vi "configuration UI.vi"() -> ()   [LabVIEW 2013, in "UI Reference editor node.lvclass"]
uses:
  UI Reference editor node.lvclass
  <vilib>/CEF_TreeControl/Node/NodeRef.ctl
  <vilib>/CEF_TreeControl/Node/NISE_CEF_Node.lvclass
  <vilib>/NI/AMC/Message Queue.ctl
  <vilib>/NI/AMC/Message.ctl
  <vilib>/NI/Tools/Keyed Array/KeyedArray.ctl
  <vilib>/CEF_TreeControl/Node/UserEventRef.ctl
  <vilib>/CEF_TreeControl/Controls/EventCluster.ctl
  module/configuration/UI Reference configuration.lvclass
  <vilib>/NI/Module Execution Interface/Engine Configuration/engine configuration.lvclass
  <vilib>/NI/Tag Bus Data Framework/Configuration Editor/Classes/Engine Parent/Engine Parent Editor Node.lvclass
  <vilib>/NI/Tag Bus/tag/tag descriptor.lvclass
  <vilib>/NI/Tag Bus/tag/Data Type.ctl
  <vilib>/NI/Tag Bus/tag/tag descriptor.lvclass/tag descriptor.ctl
  <vilib>/NI/Tag Bus Module Framework/root configuration/TBM configuration.lvclass/TBM configuration.ctl
  module/configuration/UI Reference configuration.lvclass/UI Reference configuration.ctl
  <vilib>/NI/Tag Bus/tag/write tag name.vi
  <vilib>/NI/Tag Bus/tag/write data type.vi
  <vilib>/NI/Tag Bus Module Framework/root configuration/Read instance name.vi
  module/configuration/Read VI name.vi
  <vilib>/NI/Tag Bus Data Framework/Configuration Editor/Classes/Module editor node/Read Module Configuration.vi
  <vilib>/NI/Tag Bus Module Framework/root configuration/create GUID.vi
  <vilib>/NI/Tag Bus Module Framework/root configuration/TBM configuration.lvclass
  <vilib>/NI/Tag Bus Module Framework/module configuration/TBM module configuration.lvclass
  <vilib>/NI/Tag Bus Module Framework/channel/TBM channel.lvclass
  <vilib>/CEF_TreeControl/NISE_CEF_TreeControl.lvlib
  <vilib>/NI/Tag Bus Data Framework/Configuration Editor/Classes/Module editor node/module editor node.lvclass
  <vilib>/NI/Tools/Keyed Array/Tools_KeyedArray.lvlib
  <vilib>/NI/AMC/AMC.lvlib
panel:
  in  "Tab Control":enum32{"Static Configuration"}(tab)
  in  "autogen":bool
  in  "browse":bool
  out "UI to Load":string
  in  "hidden_remove":bool
  in  "hidden_settings":bool
  in  "hidden_Add":bool
  in  "Remove Button":bool
  in  "Add Button":bool
  in  "channel":i32(listbox)
  in  "settings":bool
  in  "user event":T1
  in  "main queue":T2
  in  "node ref":T3
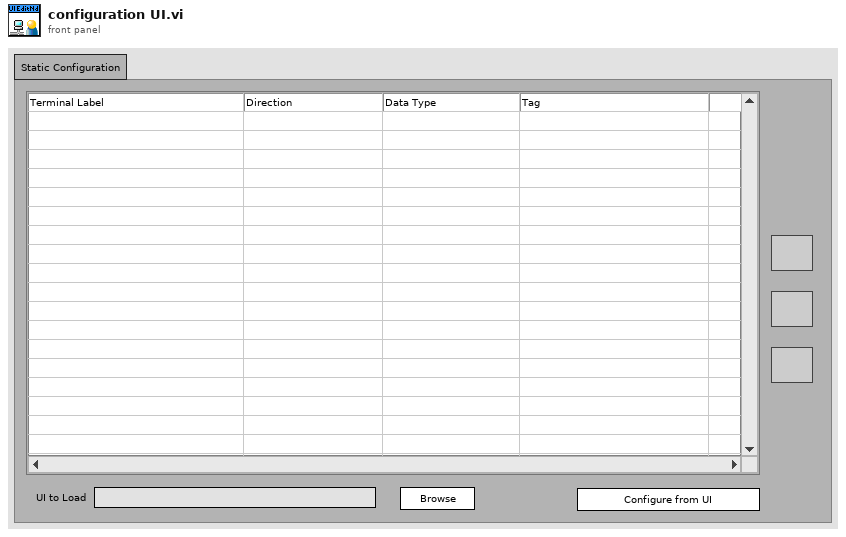
[diagram p1: front panel]
types:
  T1 = typedef "NISE_CEF_Node.lvclass/UserEventRef.ctl" = refnum<user-event>
  T2 = typedef "AMC.lvlib/Message Queue.ctl" = refnum<queue>
  T3 = typedef "NISE_CEF_Node.lvclass/NodeRef.ctl" = refnum<data-value>
  T4 = typedef "tag bus.lvlib/tag descriptor.lvclass/Data Type.ctl" = enum16{"Double", "Single", "I64", "I32", "I16", "I8", "U64", "U32", "U16", "U8", "Boolean", "String", "Array of Double", "Array of Single", "Array of I64", "Array of I32", "Array of I16", "Array of I8", "Array of U64", "Array of U32", "Array of U16", "Array of U8", "Array of Boolean", "Array of String"}
  T5 = typedef "NISE_CEF_TreeControl.lvlib/EventCluster.ctl" = cluster{"command":string, "data":string}
  T6 = typedef "UI Reference editor node.lvclass/table line.ctl" = cluster{"channel":refnum<class "TBM channel.lvclass">, "tag name":string}
  T7 = typedef "LVPoint32TypeDef.ctl" = cluster{"Horizontal":i32, "Vertical":i32}
  T8 = typedef "LVRowAndColumnTypeDef.ctl" = cluster{"Row":i32, "Column":i32}
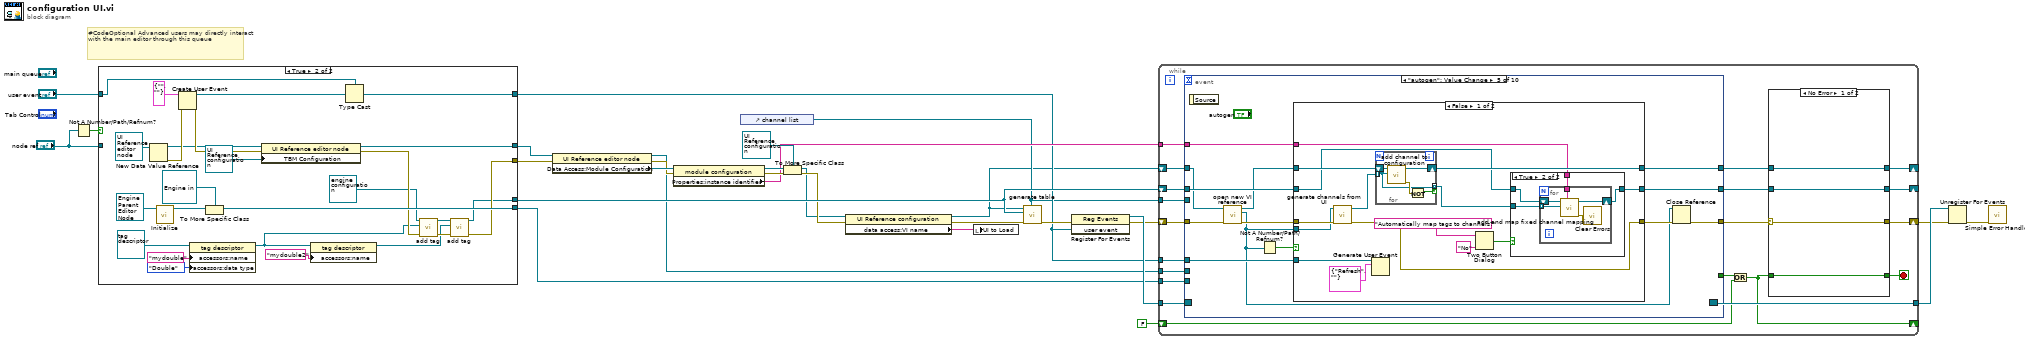
[diagram p0: block diagram]
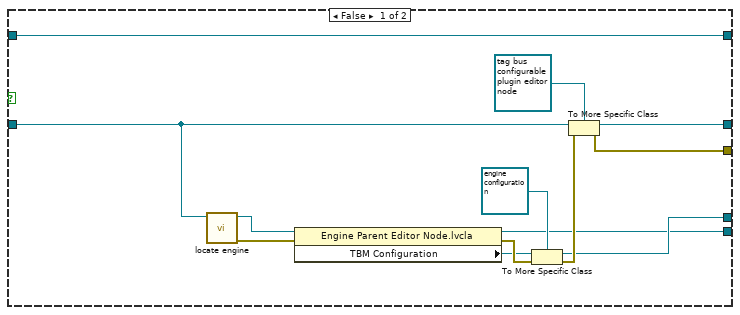
[diagram p2: hidden frame]
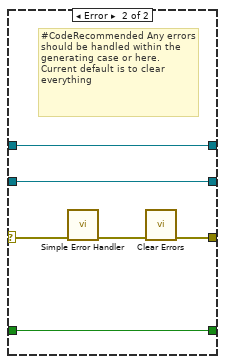
[diagram p3: hidden frame]
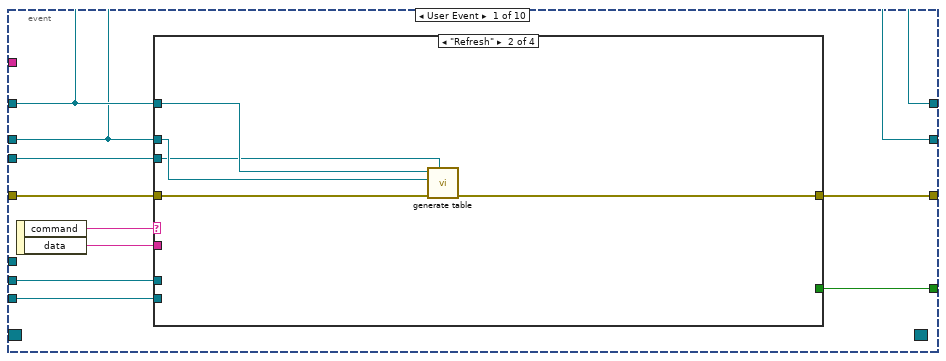
[diagram p4: hidden frame]
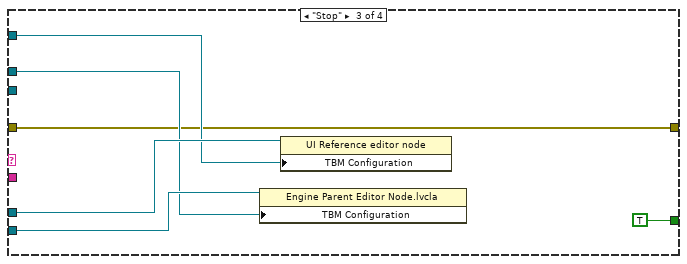
[diagram p6: hidden frame]
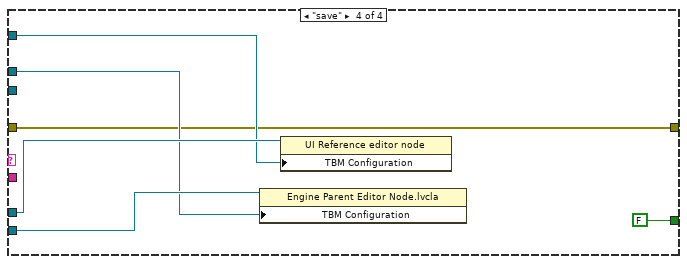
[diagram p7: hidden frame]
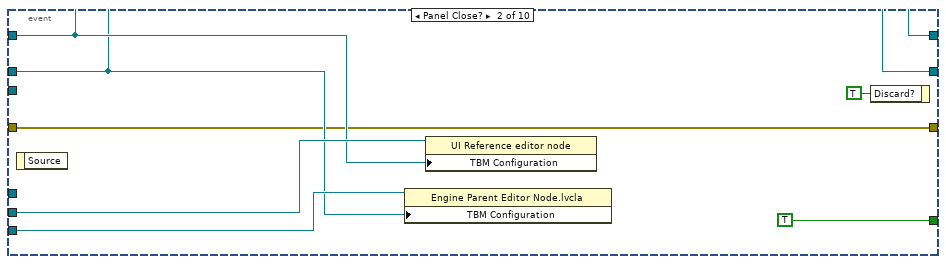
[diagram p8: hidden frame]
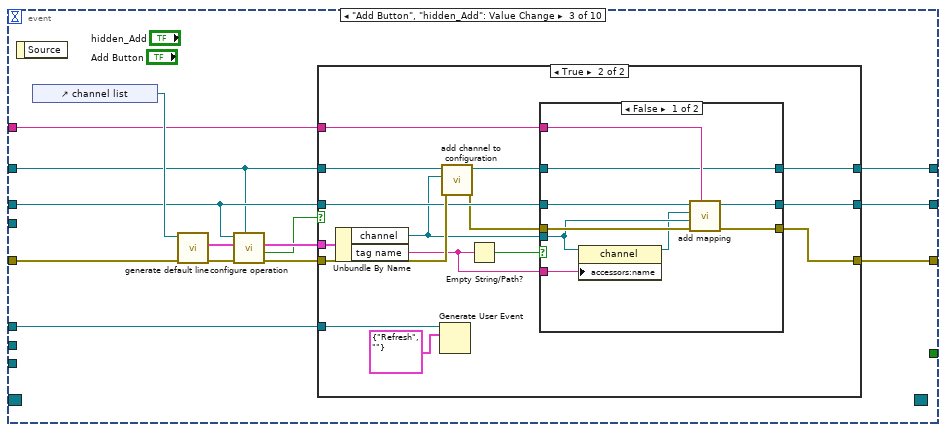
[diagram p9: hidden frame]
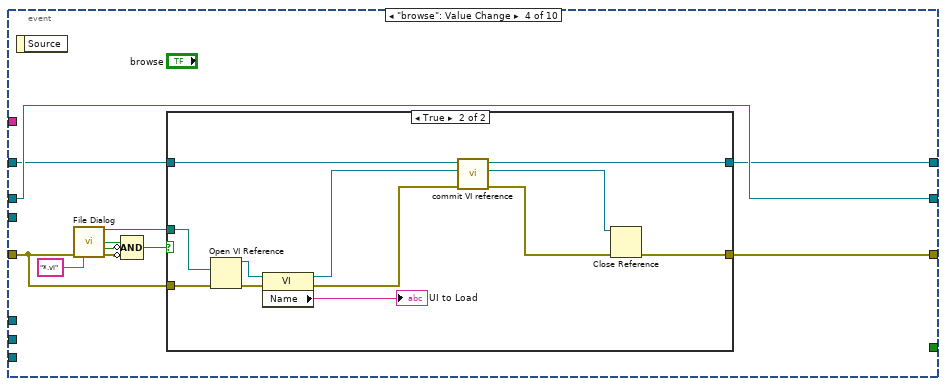
[diagram p12: hidden frame]
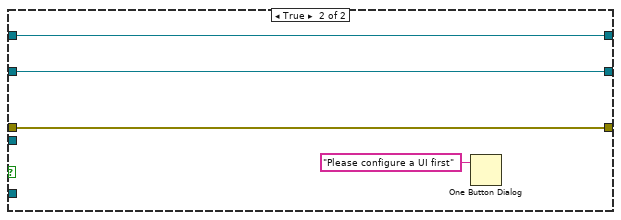
[diagram p15: hidden frame]
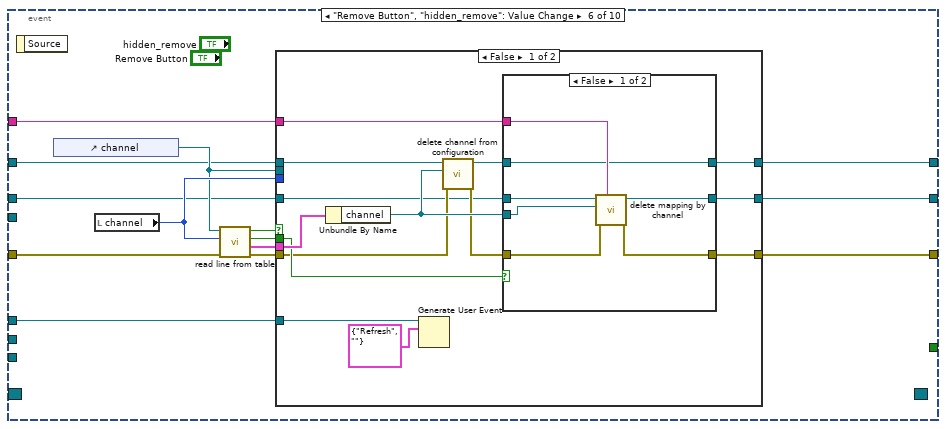
[diagram p16: hidden frame]
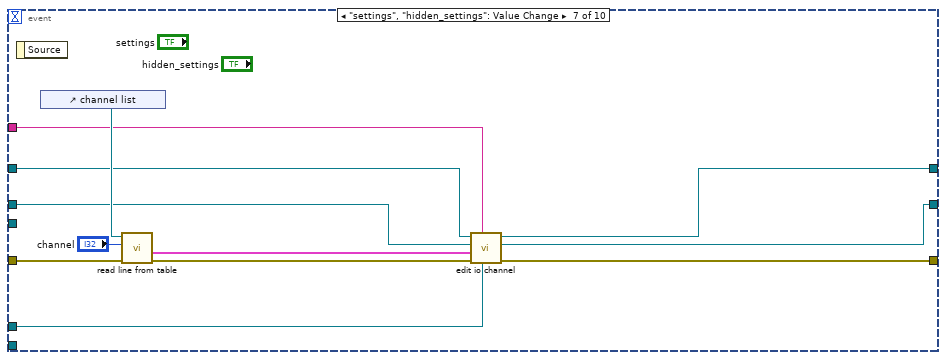
[diagram p19: hidden frame]
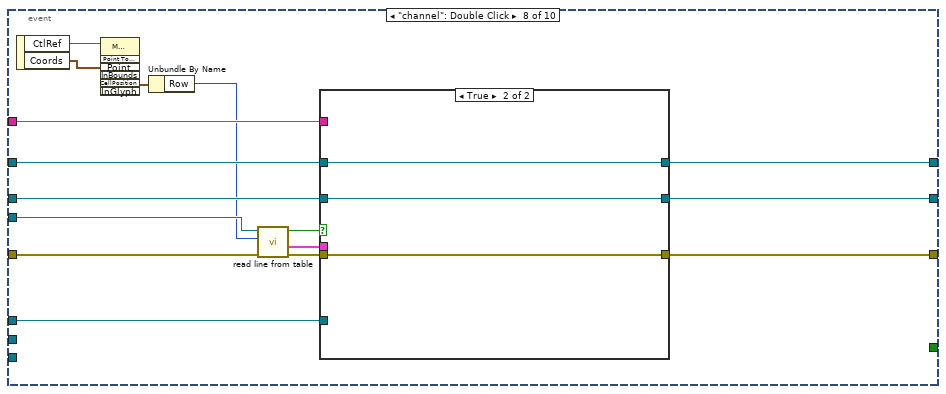
[diagram p20: hidden frame]
diagram:
  # "#CodeOptional Advanced users may directly interact with the main editor through this queue"
  n1 = Not A Number/Path/Refnum?(number/path/refnum="node ref") -> (NaN/Path/Refnum?=w19:bool)
  n2 = case shown="True" w19 {
    tunnel: "user event" -> [w41 w43]
    tunnel: [w41 w44] -> w6
    tunnel: "node ref" -> [w39 _]
    tunnel: [w38 w61] -> w12
    tunnel: [w37 w48] -> w17
    tunnel: [w30 w47] -> w14
    tunnel: [w29 w58] -> w8
    frame False {
      n3 = call <vilib>:"locate engine.vi"("component"=w39) -> ("error out"=w34:errorcluster, "engine"=w36:refnum<data-value>)  [unwired: 9 in]
      n4 = property class="Engine Parent Editor Node.lvcla"(reference=w36, error in=w34) -> (reference out=w29:refnum<data-value>, error out=w33:errorcluster, "TBM Configuration"=w32:refnum<class "TBM configuration.lvclass">)
      n5 = To More Specific Class(target class=refnum<class "engine configuration.lvclass"> refnum ("engine configuration.lvclass"), reference=w32, error in=w33) -> (specific class reference=w30:refnum<class "engine configuration.lvclass">, error out=w31:errorcluster)
      n6 = To More Specific Class(target class=refnum<data-value> refnum ("data value reference"), reference=w39, error in=w31) -> (specific class reference=w38:refnum<data-value>, error out=w37:errorcluster)
    }
    frame True {
      n7 = New Data Value Reference(data value=refnum<class "UI Reference editor node.lvclass"> refnum ("tag bus configurable plugin editor node")) -> (data value reference=w60:refnum<data-value>, error out=w63:errorcluster)  [unwired: 1 in]
      n8 = call-dynamic "Initialize.vi"("Engine in"=refnum<class "Engine Parent Editor Node.lvclass"> refnum) -> ("data value reference"=w59:T3)  [unwired: 8 in, 2 out]
      n9 = Create User Event(user event datatype=T5 {"command"="", "data"=""} ("event data"), error in=w63) -> (user event=w66:refnum<user-event>, error out=w62:errorcluster)
      n10 = property class="tag descriptor"(reference=refnum<class "tag descriptor.lvclass"> refnum ("tag descriptor"), "accessors:name"="mydouble" ("name"), "accessors:data type"=Data_Type."Double" ("data type")) -> (reference out=w45:refnum<class "tag descriptor.lvclass">)  [unwired: 1 in, 1 out]
      n11 = To More Specific Class(target class=refnum<data-value> refnum ("data value reference"), reference=w59) -> (specific class reference=w58:refnum<data-value>)  [unwired: 1 in, 1 out]
      n12 = property class="UI Reference editor node"(reference=w60, error in=w62, "TBM Configuration"=refnum<class "UI Reference configuration.lvclass"> refnum ("tag bus configurable plugin module configuration")) -> (reference out=w61:refnum<data-value>, error out=w52:errorcluster)
      n13 = property class="tag descriptor"(reference=w45, "accessors:name"="mydouble2" ("name")) -> (reference out=w46:refnum<class "tag descriptor.lvclass">)  [unwired: 1 in, 1 out]
      n14 = Type Cast(type=w43, x=w66) -> (*(type *) &x=w44:T1)
      n15 = call <vilib>:"add tag.vi"("error in"=w52, "tag descriptor"=w45, "engine configuration in"=refnum<class "engine configuration.lvclass"> refnum ("Engine Configuration")) -> ("error out"=w50:errorcluster, "engine configuration out"=w49:refnum<class "engine configuration.lvclass">)  [unwired: 7 in]
      n16 = call <vilib>:"add tag.vi"("error in"=w50, "tag descriptor"=w46, "engine configuration in"=w49) -> ("error out"=w48:errorcluster, "engine configuration out"=w47:refnum<class "engine configuration.lvclass">)  [unwired: 7 in]
    }
  }
  n17 = property class="UI Reference editor node"(reference=w12, error in=w17) -> (reference out=w9:refnum<data-value>, error out=w22:errorcluster, "Data Access:Module Configuration"=w23:refnum<class "TBM module configuration.lvclass">)
  n18 = property class="module configuration"(reference=w23, error in=w22) -> (reference out=w20:refnum<class "TBM module configuration.lvclass">, error out=w21:errorcluster, "Properties:instance identifier"=w16:string)
  n19 = control-ref of="channel list"() -> (w5:refnum<vi>)
  n20 = To More Specific Class(target class=refnum<class "UI Reference configuration.lvclass"> refnum ("tag bus configurable plugin module configuration"), reference=w20, error in=w21) -> (specific class reference=w3:refnum<class "UI Reference configuration.lvclass">, error out=w13:errorcluster)
  n21 = property class="UI Reference configuration"(reference=w3, error in=w13) -> (reference out=w2:refnum<class "UI Reference configuration.lvclass">, error out=w4:errorcluster, "data access:VI name"=w1:string)
  n22 = local write "UI to Load"(w1) -> ()
  n23 = call "generate table.vi"("table"=w5, "error in"=w4, "engine configuration"=w14, "tag bus configurable plugin module configuration"=w2) -> ("error out"=w11:errorcluster)  [unwired: 7 in]
  n24 = register-events(error in=w11, w6) -> (reference out=w28:refnum<event-registration>, error out=w10:errorcluster)  [unwired: 1 in]
  n25 = while {
    tunnel: w28 -> [w87]
    tunnel: [w86] -> w27
    shift-right: [w80] -> w26
    shift-left: w10 -> [w85]
    shift-right: [w82] -> _
    shift-left: FALSE -> [w81]
    shift-right: [w76] -> _
    shift-left: w2 -> [w79]
    shift-right: [w77] -> _
    shift-left: w14 -> [w78]
    tunnel: w16 -> [w75]
    tunnel: w9 -> [w72]
    tunnel: w8 -> [w71]
    tunnel: w6 -> [w70]
    tunnel: w5 -> [w68]
    stop <- w84 stop-if-true
    n26 = event shown="[4] \"autogen\": Value Change" {
      selector: w87 -> [_ _ _ _ _ _ _ _ _ _]
      dyn-events: [_ _ _ _ _ _ _ _ _ _] -> w86
      timeout: _ -> [_ _ _ _ _ _ _ _ _ _]
      tunnel: [w107 TRUE _ _ _ _ _ _ _ _] -> w83
      tunnel: [w99 w127 w146 w179 w203 w262 w300 w316 w330 w365] -> w69
      tunnel: w85 -> [w100 w127 w145 w181 w207 w261 w301 w317 w348 w364]
      tunnel: w79 -> [w103 w129 w133 w178 w206 w257 w294 w312 w337 w369]
      tunnel: w78 -> [w102 w128 w134 w187 w212 w256 w295 w313 w333 w368]
      tunnel: [w102 w128 w139 w187 w213 w251 w292 w310 w334 w366] -> w74
      tunnel: [w103 w129 w138 w177 w211 w250 w293 w311 w335 w367] -> w73
      tunnel: w75 -> [_ _ w137 _ w209 w252 w291 w309 _ _]
      tunnel: w72 -> [w105 w131 _ _ _ _ _ _ _ _]
      tunnel: w71 -> [w104 w130 _ _ _ _ _ _ _ _]
      tunnel: w70 -> [_ _ w135 _ w208 w249 w290 w308 _ _]
      tunnel: w68 -> [w98 _ _ _ _ _ _ w307 _ _]
      event User Event {
        n27 = event-data() -> ("command"=w106:string, "data"=w101:string)  [unwired: 1 in]
        n28 = case shown="\"Refresh\"" w106 {
          tunnel: [_ _ TRUE FALSE] -> w107
          tunnel: w105 -> [_ _ w118 w124]
          tunnel: w104 -> [_ _ w117 w123]
          tunnel: w103 -> [_ w113 w116 w122]
          tunnel: w102 -> [_ w112 w115 w121]
          tunnel: w101 -> [_ _ _ _]
          tunnel: w100 -> [w108 w111 w114 w120]
          tunnel: [w108 w110 w114 w120] -> w99
          tunnel: w98 -> [_ w109 _ _]
          frame Default {
          }
          frame "Refresh" {
            n29 = call "generate table.vi"("table"=w109, "error in"=w111, "engine configuration"=w112, "tag bus configurable plugin module configuration"=w113) -> ("error out"=w110:errorcluster)  [unwired: 7 in]
          }
          frame "Stop" {
            n30 = property class="Engine Parent Editor Node.lvcla"(reference=w117, "TBM Configuration"=w115) -> ()  [unwired: 1 in, 2 out]
            n31 = property class="UI Reference editor node"(reference=w118, "TBM Configuration"=w116) -> ()  [unwired: 1 in, 2 out]
          }
          frame "save" {
            n32 = property class="Engine Parent Editor Node.lvcla"(reference=w123, "TBM Configuration"=w121) -> ()  [unwired: 1 in, 2 out]
            n33 = property class="UI Reference editor node"(reference=w124, "TBM Configuration"=w122) -> ()  [unwired: 1 in, 2 out]
          }
        }
      }
      event Panel Close? {
        n34 = event-data() -> ()  [unwired: 1 in, 1 out]
        n35 = property class="Engine Parent Editor Node.lvcla"(reference=w130, "TBM Configuration"=w128) -> ()  [unwired: 1 in, 2 out]
        n36 = property class="UI Reference editor node"(reference=w131, "TBM Configuration"=w129) -> ()  [unwired: 1 in, 2 out]
        n37 = event-data("Discard?"=TRUE) -> ()  [unwired: 1 in, 1 out]
      }
      event "Add Button", "hidden_Add": Value Change {
        n38 = event-data() -> ()  [unwired: 1 in, 1 out]
        n39 = control-ref of="channel list"() -> (w144:refnum<vi>)
        n40 = call "generate default line.vi"("error in"=w145, "operations table"=w144) -> ("error out"=w142:errorcluster, "line"=w143:T6)  [unwired: 8 in]
        n41 = call "configure operation.vi"("tag bus configurable plugin module configuration"=w133, "error in"=w142, "line item in"=w143, "engine configuration"=w134) -> ("error out"=w140:errorcluster, "success"=w136:bool, "line item out"=w141:T6)  [unwired: 4 in, 1 out]
        n42 = case shown="True" w136 {
          tunnel: [w149 w152] -> w146
          tunnel: w140 -> [w149 w162]
          tunnel: w134 -> [w148 w160]
          tunnel: w141 -> [_ w163]
          tunnel: w133 -> [w147 w164]
          tunnel: [w148 w159] -> w139
          tunnel: [w147 w153] -> w138
          tunnel: w137 -> [_ w156]
          tunnel: w135 -> [_ w151]
          frame False {
          }
          frame True {
            n43 = Unbundle By Name(w163) -> ("channel"=w157:refnum<class "TBM channel.lvclass">, "tag name"=w155:string)
            n44 = Generate User Event(user event=w151, event data cluster=T5 {"command"="Refresh", "data"=""} ("event data")) -> ()  [unwired: 2 in, 2 out]
            n45 = call "add channel to configuration.vi"("error in"=w162, "channel"=w157, "UI Reference configuration in"=w164) -> ("error out"=w158:errorcluster, "UI Reference configuration out"=w154:refnum<class "UI Reference configuration.lvclass">)  [unwired: 7 in]
            n46 = Empty String/Path?(string/path=w155) -> (empty?=w161:bool)
            n47 = case shown="False" w161 {
              tunnel: w160 -> [w173 w176]
              tunnel: [w172 w176] -> w159
              tunnel: w158 -> [w171 w175]
              tunnel: w157 -> [w169 _]
              tunnel: w156 -> [w170 _]
              tunnel: w155 -> [w168 _]
              tunnel: [w166 w175] -> w152
              tunnel: w154 -> [w165 w174]
              tunnel: [w165 w174] -> w153
              frame False {
                n48 = property class="channel"(reference=w169, "accessors:name"=w168) -> (reference out=w167:refnum<class "TBM channel.lvclass">)  [unwired: 1 in, 1 out]
                n49 = call <vilib>:"add mapping.vi"("owner ID"=w170, "error in"=w171, "channel"=w169, "tag descriptor"=w167, "engine configuration"=w173) -> ("error out"=w166:errorcluster, "engine configuration out"=w172:refnum<class "engine configuration.lvclass">)  [unwired: 5 in]
              }
              frame True {
              }
            }
          }
        }
      }
      event "browse": Value Change {
        n50 = event-data() -> ()  [unwired: 1 in, 1 out]
        n51 = call "File Dialog"("error in"=w181, "pattern (all files)"="*.vi") -> ("selected path"=w180:path, "exists"=w185:bool, "cancelled"=w184:bool, "error out"=w183:errorcluster)  [unwired: 10 in]
        n52 = Compound Arithmetic op=AND(w185, invert w184, invert w183) -> (w182:bool)
        n53 = case shown="True" w182 {
          tunnel: w181 -> [w189 w201]
          tunnel: w180 -> [_ w200]
          tunnel: [w189 w193] -> w179
          tunnel: w178 -> [w188 w196]
          tunnel: [w188 w195] -> w177
          frame False {
          }
          frame True {
            n54 = Open VI Reference(vi path=w200, error in (no error)=w201) -> (vi reference=w198:refnum<vi>, error out=w199:errorcluster)  [unwired: 4 in]
            n55 = property class="VI"(reference=w198, error in=w199) -> (reference out=w190:refnum<vi>, error out=w191:errorcluster, "Name"=→"UI to Load":string)
            n56 = call "commit VI reference.vi"("error in"=w191, "VI Refnum in"=w190, "UI Reference configuration in"=w196) -> ("error out"=w194:errorcluster, "VI Refnum out"=w192:refnum<vi>, "UI Reference configuration out"=w195:refnum<class "UI Reference configuration.lvclass">)  [unwired: 6 in]
            n57 = Close Reference(reference=w192, error in (no error)=w194) -> (error out=w193:errorcluster)
          }
        }
      }
      event "autogen": Value Change {
        n58 = event-data() -> ()  [unwired: 1 in, 1 out]
        n59 = call "open new VI reference.vi"("error in"=w207, "UI Reference configuration in"=w206) -> ("error out"=w204:errorcluster, "VI Refnum"=w202:refnum<vi>, "UI Reference configuration out"=w205:refnum<class "UI Reference configuration.lvclass">)  [unwired: 7 in]
        n60 = Not A Number/Path/Refnum?(number/path/refnum=w202) -> (NaN/Path/Refnum?=w214:bool)
        n61 = case shown="False" w214 {
          tunnel: w204 -> [w229 w246]
          tunnel: w205 -> [w227 w247]
          tunnel: [w220 w248] -> w213
          tunnel: w212 -> [w221 w248]
          tunnel: [w222 w247] -> w211
          tunnel: [w218 w246] -> w210
          tunnel: w202 -> [w228 _]
          tunnel: w209 -> [w217 _]
          tunnel: w208 -> [w215 _]
          frame False {
            n62 = call "generate channels from UI.vi"("error in"=w229, "VI Refnum"=w228) -> ("error out"=w218:errorcluster, "channels"=w226:refnum<class "TBM channel.lvclass">[])  [unwired: 8 in]
            n63 = Generate User Event(user event=w215, event data cluster=T5 {"command"="Refresh", "data"=""} ("event data")) -> ()  [unwired: 2 in, 2 out]
            n64 = for {
              tunnel: w226 -> [w241] mode=indexing
              shift-right: [w243] -> w222
              shift-left: w227 -> [w244]
              tunnel: [w241] -> w219 mode=indexing if=w240
              n65 = call "add channel to configuration.vi"("channel"=w241, "UI Reference configuration in"=w244) -> ("error out"=w242:errorcluster, "UI Reference configuration out"=w243:refnum<class "UI Reference configuration.lvclass">)  [unwired: 8 in]
              n66 = Not(x=w242) -> (.not. x?=w240:bool)
            }
            n67 = Two Button Dialog(message="Automatically map tags to channels?", 1:"No" ("F button name (\"Cancel\")")) -> (T button?=w223:bool)  [unwired: 1 in]
            n68 = case shown="True" w223 {
              tunnel: w221 -> [w230 w234]
              tunnel: [w230 w233] -> w220
              tunnel: w219 -> [_ w232]
              tunnel: w217 -> [_ w231]
              frame False {
              }
              frame True {
                n69 = for {
                  shift-right: [w238] -> w233
                  shift-left: w234 -> [w239]
                  tunnel: w232 -> [w237] mode=indexing
                  tunnel: w231 -> [w235]
                  n70 = call <vilib>:"add and map fixed channel mapping.vi"("module instance"=w235, "fixed channel"=w237, "engine configuration in"=w239) -> ("error out"=w236:errorcluster, "engine configuration out"=w238:refnum<class "engine configuration.lvclass">)  [unwired: 7 in]
                  n71 = call <vilib>:"Clear Errors.vi"("error in (no error)"=w236) -> ()  [unwired: 6 in, 1 out]
                }
              }
            }
          }
          frame True {
            n72 = One Button Dialog(message="Please configure a UI first") -> ()  [unwired: 1 in, 1 out]
          }
        }
        n73 = Close Reference(reference=w202, error in (no error)=w210) -> (error out=w203:errorcluster)
      }
      event "Remove Button", "hidden_remove": Value Change {
        n74 = event-data() -> ()  [unwired: 1 in, 1 out]
        n75 = control-ref of="channel"() -> (w259:refnum<vi>)
        n76 = local read "channel"() -> (w260:i32)
        n77 = call "read line from table.vi"("error in"=w261, "line number"=w260, "channels table"=w259) -> ("error out"=w253:errorcluster, "line"=w258:T6, "empty tag?"=w254:bool, "empty channel?"=w255:bool)  [unwired: 5 in]
        n78 = case shown="False" w255 {
          tunnel: [w265 w288] -> w262
          tunnel: w260 -> [_ _]
          tunnel: w259 -> [_ _]
          tunnel: w258 -> [w276 _]
          tunnel: w257 -> [w274 w287]
          tunnel: w256 -> [w269 w289]
          tunnel: w254 -> [w275 _]
          tunnel: w253 -> [w272 w288]
          tunnel: w252 -> [w268 _]
          tunnel: [w267 w289] -> w251
          tunnel: [w266 w287] -> w250
          tunnel: w249 -> [w263 _]
          frame False {
            n79 = Unbundle By Name(w276) -> ("channel"=w273:refnum<class "TBM channel.lvclass">)
            n80 = Generate User Event(user event=w263, event data cluster=T5 {"command"="Refresh", "data"=""} ("event data")) -> ()  [unwired: 2 in, 2 out]
            n81 = call "delete channel from configuration.vi"("error in"=w272, "channel"=w273, "UI Reference configuration in"=w274) -> ("error out"=w270:errorcluster, "UI Reference configuration out"=w271:refnum<class "UI Reference configuration.lvclass">)  [unwired: 7 in]
            n82 = case shown="False" w275 {
              tunnel: w273 -> [w282 _]
              tunnel: w271 -> [w277 w284]
              tunnel: w270 -> [w280 w285]
              tunnel: w269 -> [w283 w286]
              tunnel: w268 -> [w281 _]
              tunnel: [w279 w286] -> w267
              tunnel: [w278 w285] -> w265
              tunnel: [w277 w284] -> w266
              frame False {
                n83 = call <vilib>:"delete mapping by channel.vi"("owner ID"=w281, "error in"=w280, "channel"=w282, "engine configuration in"=w283) -> ("error out"=w278:errorcluster, "engine configuration out"=w279:refnum<class "engine configuration.lvclass">)  [unwired: 6 in]
              }
              frame True {
              }
            }
          }
          frame True {
          }
        }
      }
      event "settings", "hidden_settings": Value Change {
        n84 = event-data() -> ()  [unwired: 1 in, 1 out]
        n85 = control-ref of="channel list"() -> (w299:refnum<vi>)
        n86 = call "read line from table.vi"("error in"=w301, "line number"="channel", "channels table"=w299) -> ("error out"=w298:errorcluster, "line"=w297:T6)  [unwired: 5 in, 2 out]
        n87 = call "edit io channel.vi"("user event"=w290, "Properties:instance identifier"=w291, "error in"=w298, "line"=w297, "engine configuration in"=w295, "tag bus configurable plugin module configuration in"=w294) -> ("error out"=w300:errorcluster, "engine configuration"=w292:refnum<class "engine configuration.lvclass">, "tag bus configurable plugin module configuration out"=w293:refnum<class "UI Reference configuration.lvclass">)  [unwired: 3 in]
      }
      event "channel": Double Click {
        n88 = event-data() -> ("CtlRef"=w306:refnum<vi>, "Coords"=w305:T7)  [unwired: 1 in]
        n89 = invoke class="MCListbox (strict)" method="Point To Row Column"(reference=w306, "Point"=w305) -> ("CellPosition"=w304:T8)  [unwired: 5 in, 6 out]
        n90 = Unbundle By Name(w304) -> ("Row"=w303:i32)
        n91 = call "read line from table.vi"("error in"=w317, "line number"=w303, "channels table"=w307) -> ("error out"=w315:errorcluster, "line"=w314:T6, "empty channel?"=w302:bool)  [unwired: 5 in, 1 out]
        n92 = case shown="True" w302 {
          tunnel: [w326 w327] -> w316
          tunnel: w315 -> [w325 w327]
          tunnel: w314 -> [w324 _]
          tunnel: w313 -> [w323 w328]
          tunnel: w312 -> [w322 w329]
          tunnel: [w321 w329] -> w311
          tunnel: [w320 w328] -> w310
          tunnel: w309 -> [w319 _]
          tunnel: w308 -> [w318 _]
          frame False {
            n93 = call "edit io channel.vi"("user event"=w318, "Properties:instance identifier"=w319, "error in"=w325, "line"=w324, "engine configuration in"=w323, "tag bus configurable plugin module configuration in"=w322) -> ("error out"=w326:errorcluster, "engine configuration"=w320:refnum<class "engine configuration.lvclass">, "tag bus configurable plugin module configuration out"=w321:refnum<class "UI Reference configuration.lvclass">)  [unwired: 3 in]
          }
          frame True {
          }
        }
      }
      event "channel": Shortcut Menu Activation? {
        n94 = event-data() -> ("MenuRef"=w344:refnum<k9>, "CtlRef"=w346:refnum<vi>, "Coords"=w345:T7)  [unwired: 1 in]
        n95 = invoke class="MCListbox (strict)" method="Point To Row Column"(reference=w346, "Point"=w345) -> (reference out=w343:refnum<vi>, error out=w342:errorcluster, "CellPosition"=w341:T8)  [unwired: 5 in, 4 out]
        n96 = Delete Menu Items(6:w348, 9:w344) -> (0:w331:errorcluster, 3:w332:refnum<k9>)  [unwired: 2 in]
        n97 = Unbundle(w341) -> ("Row"=w339:i32)  [unwired: 1 out]
        n98 = property class="MCListbox (strict)"(reference=w343, error in=w342) -> ("ItemNames"=w340:string[][])  [unwired: 2 out]
        n99 = Index Array(array=w340, index (row)=w339, index (col)=0 ("disabled index (col)")) -> (element=w336:string)
        n100 = case shown="\"\"" w336 {
          tunnel: w337 -> [w354 w360]
          tunnel: [w354 w360] -> w335
          tunnel: [w353 w359] -> w334
          tunnel: w333 -> [w353 w359]
          tunnel: w332 -> [w352 w358]
          tunnel: w331 -> [w351 w357]
          tunnel: [w350 w356] -> w330
          frame Default {
            w349 = string[] ["Add", "Edit", "Delete"] ("item names")
            n101 = Insert Menu Items(6:w351, 7:w349, 8:w349, 9:w352) -> (0:w350:errorcluster)  [unwired: 2 in, 2 out]
          }
          frame "" {
            w355 = string[] ["Add"] ("item names")
            n102 = Insert Menu Items(6:w357, 7:w355, 8:w355, 9:w358) -> (0:w356:errorcluster)  [unwired: 2 in, 2 out]
          }
        }
        n103 = event-data("Discard?"=FALSE) -> ()  [unwired: 1 in, 1 out]
      }
      event "channel": Shortcut Menu Selection (User) {
        n104 = event-data() -> ("ItemTag"=w370:string, "CtlRef"=w371:refnum<vi>, "Coords"=w372:T7)  [unwired: 1 in]
        n105 = invoke class="MCListbox (strict)" method="Point To Row Column"(reference=w371, "Point"=w372) -> ("CellPosition"=w362:T8)  [unwired: 5 in, 6 out]
        n106 = Unbundle By Name(w362) -> ("Row"=w361:i32)
        n107 = property on="channel" class="MCListbox (strict)"(error in=w364, "Value"=w361) -> (error out=w363:errorcluster)  [unwired: 1 in, 1 out]
        n108 = case shown="\"Delete\"" w370 {
          tunnel: w363 -> [w373 w377 w383 w388]
          tunnel: w369 -> [w375 w380 w385 w390]
          tunnel: w368 -> [w374 w379 w384 w389]
          tunnel: [w375 w380 w385 w390] -> w367
          tunnel: [w374 w379 w384 w389] -> w366
          tunnel: [w373 w376 w382 w387] -> w365
          frame Default {
          }
          frame "Add" {
            n109 = property on="hidden_Add" class="Bool (strict)"(error in=w377, "Val(Sgnl)"=TRUE ("Value (Signaling)")) -> (error out=w376:errorcluster)  [unwired: 1 in, 1 out]
          }
          frame "Edit" {
            n110 = property on="hidden_settings" class="Bool (strict)"(error in=w383, "Val(Sgnl)"=TRUE ("Value (Signaling)")) -> (error out=w382:errorcluster)  [unwired: 1 in, 1 out]
          }
          frame "Delete" {
            n111 = property on="hidden_remove" class="Bool (strict)"(error in=w388, "Val(Sgnl)"=FALSE ("Value (Signaling)")) -> (error out=w387:errorcluster)  [unwired: 1 in, 1 out]
          }
        }
      }
    }
    n112 = Or(x=w83, y=w81) -> (x .or. y?=w82:bool)
    n113 = case shown="No Error" w69 {
      selector: w69 -> [w88 w96]
      tunnel: [w91 w97] -> w84
      tunnel: w82 -> [w91 w97]
      tunnel: [w88 w94] -> w80
      tunnel: w74 -> [w89 w93]
      tunnel: [w89 w93] -> w77
      tunnel: w73 -> [w90 w92]
      tunnel: [w90 w92] -> w76
      frame No Error {
      }
      frame Error {
        # "#CodeRecommended Any errors should be handled within the generating case or here. Current default is to clear everything"
        n114 = call <vilib>:"Simple Error Handler.vi"("error in (no error)"=w96) -> ("error out"=w95:errorcluster)  [unwired: 4 in, 4 out]
        n115 = call <vilib>:"Clear Errors.vi"("error in (no error)"=w95) -> ("error out"=w94:errorcluster)  [unwired: 6 in]
      }
    }
  }
  n116 = Unregister For Events(event registration refnum=w27, error in=w26) -> (error out=w7:errorcluster)
  n117 = call <vilib>:"Simple Error Handler.vi"("error in (no error)"=w7) -> ()  [unwired: 4 in, 5 out]
